vi "Clear leds (SubVI).vi"(11 "Boolean refs":refnum<vi>[](array[refnum])) -> (3 "Boolean refs out":refnum<vi>[](array[refnum]))   [LabVIEW 2021]
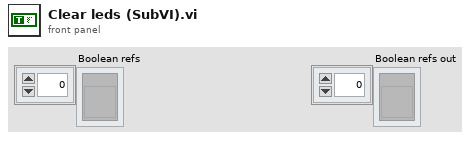
[diagram p1: front panel]
types:
  T1 = cluster{"accent s color":u32, "accent s color":u32}
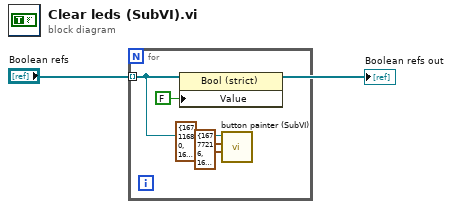
[diagram p0: block diagram]
diagram:
  n1 = for {
    tunnel: "Boolean refs" -> [w4] mode=indexing
    n2 = property class="Bool (strict)"(reference=w4, "Value"=FALSE) -> ()  [unwired: 1 in, 2 out]
    n3 = call "button painter (SubVI).vi"("Off state"=cluster{"accent color":u32, "accent color":u32} {"accent color"=16777216, "accent color"=16777216}, "On state"=T1 {"accent s color"=16711680, "accent s color"=16711680}, "Button ref in"=w4) -> ()  [unwired: 9 in]
  }
  "Boolean refs out" <- "Boolean refs"
